vi "HumanNetwork.vi"(8 "error in (no error)":errorcluster) -> (0 "error out":errorcluster)   [LabVIEW 2023]
doc: "Human Network\n\nInput\n --Error in \n\nOutput\n --Error out"
uses:
  HumanGlobal.vi
  <vilib>/Rock Robotics/Network Tables/NT Write Number.vi
  <vilib>/Rock Robotics/Network Tables/NT Write Boolean.vi
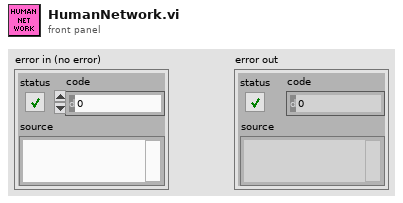
[diagram p1: front panel]
types:
  T1 = typedef "HumanDriveModeENUM.ctl" = enum16{"0 - Normal Swerve", "1 - Auto traj  - Left Speaker", "2 - Auto traj - Center Speaker", "3 - Auto traj - Speaker Right", "4 - Auto traj - Amp", "5 - Auto traj - Source", "6 - Auto traj -  Left Stage", "7 - Auto traj - Center Stage", "8 - Auto traj - Right Stage"}
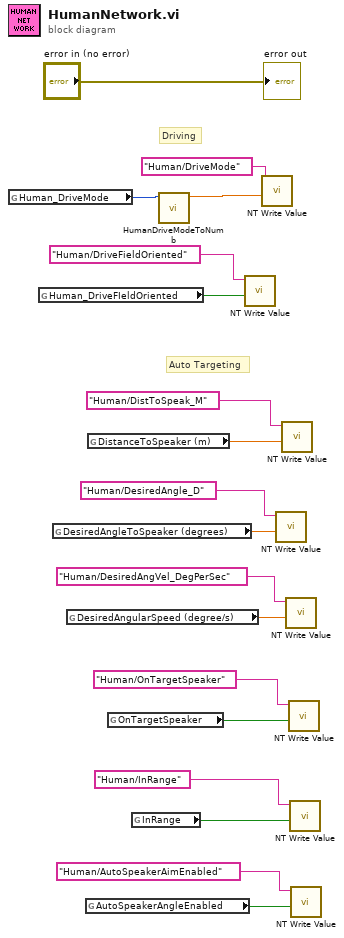
[diagram p0: block diagram]
diagram:
  # "Auto Targeting"
  # "Driving"
  n1 = global read "HumanGlobal.vi" "Human_DriveMode"() -> (w16:T1)
  n2 = global read "HumanGlobal.vi" "Human_DriveFIeldOriented"() -> (w13:bool)
  n3 = global read "HumanGlobal.vi" "DesiredAngleToSpeaker (degrees)"() -> (w9:dbl)
  n4 = global read "HumanGlobal.vi" "DesiredAngularSpeed (degree/s)"() -> (w7:dbl)
  n5 = global read "HumanGlobal.vi" "AutoSpeakerAngleEnabled"() -> (w1:bool)
  n6 = global read "HumanGlobal.vi" "DistanceToSpeaker (m)"() -> (w11:dbl)
  n7 = global read "HumanGlobal.vi" "OnTargetSpeaker"() -> (w5:bool)
  n8 = global read "HumanGlobal.vi" "InRange"() -> (w3:bool)
  n9 = call "HumanDriveModeToNumb.vi"("Human_DriveMode"=w16) -> ("StateNumber"=w15:dbl)  [unwired: 10 in]
  n10 = call-poly <vilib>:"NT Write Value.vi"("value"=w13, "name"="Human/DriveFieldOriented") -> ()  [unwired: 9 in, 1 out]
  n11 = call-poly <vilib>:"NT Write Value.vi"("value"=w15, "name"="Human/DriveMode") -> ()  [unwired: 9 in, 1 out]
  n12 = call-poly <vilib>:"NT Write Value.vi"("value"=w9, "name"="Human/DesiredAngle_D") -> ()  [unwired: 9 in, 1 out]
  n13 = call-poly <vilib>:"NT Write Value.vi"("value"=w11, "name"="Human/DistToSpeak_M") -> ()  [unwired: 9 in, 1 out]
  n14 = call-poly <vilib>:"NT Write Value.vi"("value"=w7, "name"="Human/DesiredAngVel_DegPerSec") -> ()  [unwired: 9 in, 1 out]
  n15 = call-poly <vilib>:"NT Write Value.vi"("value"=w5, "name"="Human/OnTargetSpeaker") -> ()  [unwired: 9 in, 1 out]
  n16 = call-poly <vilib>:"NT Write Value.vi"("value"=w3, "name"="Human/InRange") -> ()  [unwired: 9 in, 1 out]
  n17 = call-poly <vilib>:"NT Write Value.vi"("value"=w1, "name"="Human/AutoSpeakerAimEnabled") -> ()  [unwired: 9 in, 1 out]
  "error out" <- "error in (no error)"
